vi "ListNormalDeviceClasses.vi"() -> (0 "Detected Device Classes":T1(array[cluster]))   [LabVIEW 2013]
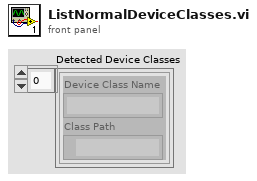
[diagram p1: front panel]
types:
  T1 = cluster{"Device Class Name":string, "Class Path":path}[]
  T2 = cluster{"Device Class Name":string, "Class Path":path}
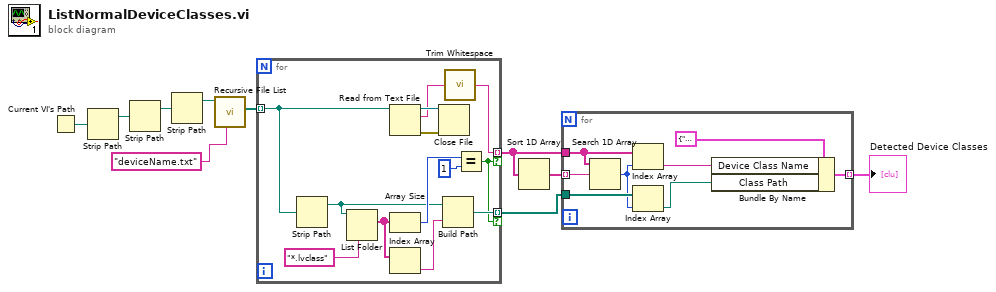
[diagram p0: block diagram]
diagram:
  n1 = Current VI's Path() -> (path=w10:path)
  n2 = Strip Path(path=w10) -> (stripped path=w4:path)  [unwired: 1 out]
  n3 = Strip Path(path=w4) -> (stripped path=w3:path)  [unwired: 1 out]
  n4 = Strip Path(path=w3) -> (stripped path=w2:path)  [unwired: 1 out]
  n5 = call <vilib>:"Recursive File List.vi"("pattern"="deviceName.txt", "Folder Path"=w2) -> ("All Files in Dir"=w8:path[])  [unwired: 5 in, 4 out]
  n6 = for {
    tunnel: w8 -> [w19] mode=indexing
    tunnel: [w20] -> w6 mode=indexing if=w11
    tunnel: [w12] -> w5 mode=indexing if=w11
    n7 = Strip Path(path=w19) -> (stripped path=w13:path)  [unwired: 1 out]
    n8 = List Folder(path=w13, pattern="*.lvclass") -> (filenames=w15:string[])  [unwired: 2 in, 3 out]
    n9 = Read from Text File(file (use dialog)=w19) -> (refnum out=w22:refnum<file>, text=w21:string, error out=w23:errorcluster)  [unwired: 3 in, 1 out]
    n10 = Array Size(array=w15) -> (size(s)=w16:i32)
    n11 = Index Array(array=w15) -> (element=w14:string)  [unwired: 1 in]
    n12 = Close File(refnum=w22, error in=w23) -> ()  [unwired: 2 out]
    n13 = Build Path(base path=w13, name or relative path=w14) -> (appended path=w12:path)
    n14 = call <vilib>:"Trim Whitespace.vi"("string"=w21) -> ("trimmed string"=w20:string)  [unwired: 1 in]
    n15 = Equal?(x=w16, y=1) -> (x = y?=w11:bool)
  }
  n16 = Sort 1D Array(array=w6) -> (sorted array=w7:string[])
  n17 = for {
    tunnel: w7 -> [w31] mode=indexing
    tunnel: w6 -> [w28]
    tunnel: w5 -> [w30]
    tunnel: [w24] -> w1 mode=indexing
    n18 = Search 1D Array(1D array=w28, element=w31) -> (index of element=w29:i32)  [unwired: 1 in]
    n19 = Index Array(array=w28, index=w29) -> (element=w26:string)
    n20 = Index Array(array=w30, index=w29) -> (element=w25:path)
    n21 = Bundle By Name(cluster=T2 {"Device Class Name"="", "Class Path"=path ""} ("Chosen Device"), "Device Class Name"=w26, "Class Path"=w25) -> (w24:T2)
  }
  "Detected Device Classes" <- w1
